vi "Check if Using Pixel Fonts.vi"(10 "desired font(Application)":T2(ring), 11 "[user-specified font]":T1) -> (3 "use_pixel_fonts":bool)   [LabVIEW 2021, in "Picture Pixel Fonts.lvlib"]
uses:
  <vilib>/LabVIEW Icon API/Pixel Fonts/Picture Pixel Fonts.lvlib
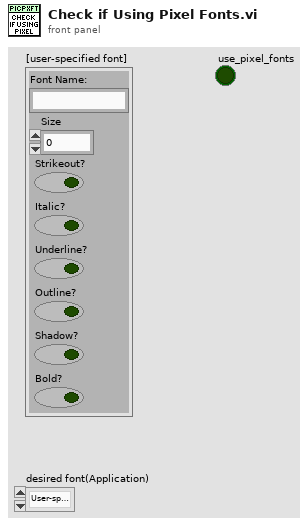
[diagram p1: front panel]
types:
  T1 = cluster{"Font Name:":string, "Size":i16, "Strikeout?":bool, "Italic?":bool, "Underline?":bool, "Outline?":bool, "Shadow?":bool, "Bold?":bool}
  T2 = enum16{"User-specified Font", "Application Font", "System Font", "Dialog Font"}
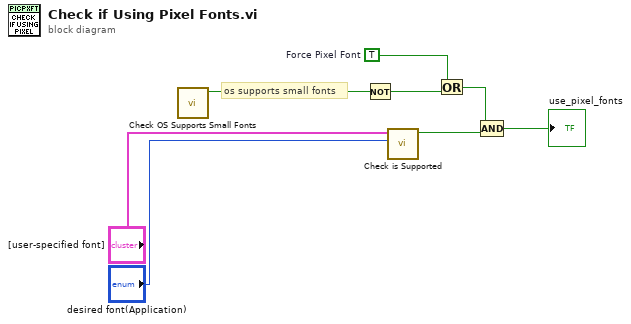
[diagram p0: block diagram]
diagram:
  w3 = TRUE  # Force Pixel Font
  # "os supports small fonts"
  n1 = call <vilib>:"Check OS Supports Small Fonts.vi"() -> ("os_supports_small_fonts"=w4:bool)  [unwired: 11 in]
  n2 = Not(x=w4) -> (.not. x?=w7:bool)
  n3 = call <vilib>:"Check is Supported.vi"("desired font(Application)"="desired font(Application)", "[user-specified font]"="[user-specified font]") -> ("is_supported"=w6:bool)  [unwired: 9 in]
  n4 = Or(x=w3, y=w7) -> (x .or. y?=w5:bool)
  n5 = Compound Arithmetic op=AND(w5, w6) -> (→"use_pixel_fonts":bool)
